vi "Optics_Open_COM.VI"(8 "Error in":errorcluster, 11 "VISA in":refnum<visa-resource-name>) -> (0 "Error out":errorcluster, 3 "VISA out":refnum<visa-resource-name>)   [LabVIEW 2021]
uses:
  <vilib>/Instr/_visa.llb/VISA Configure Serial Port (Instr).vi
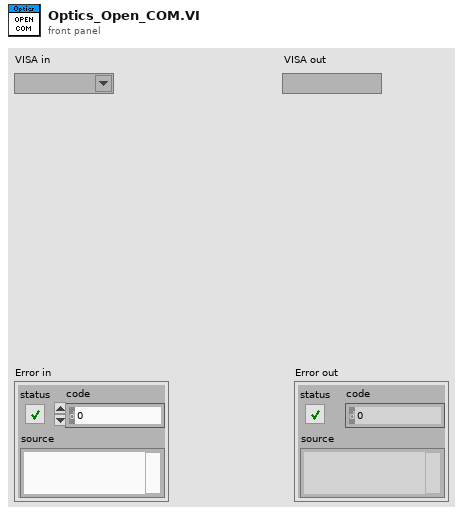
[diagram p1: front panel]
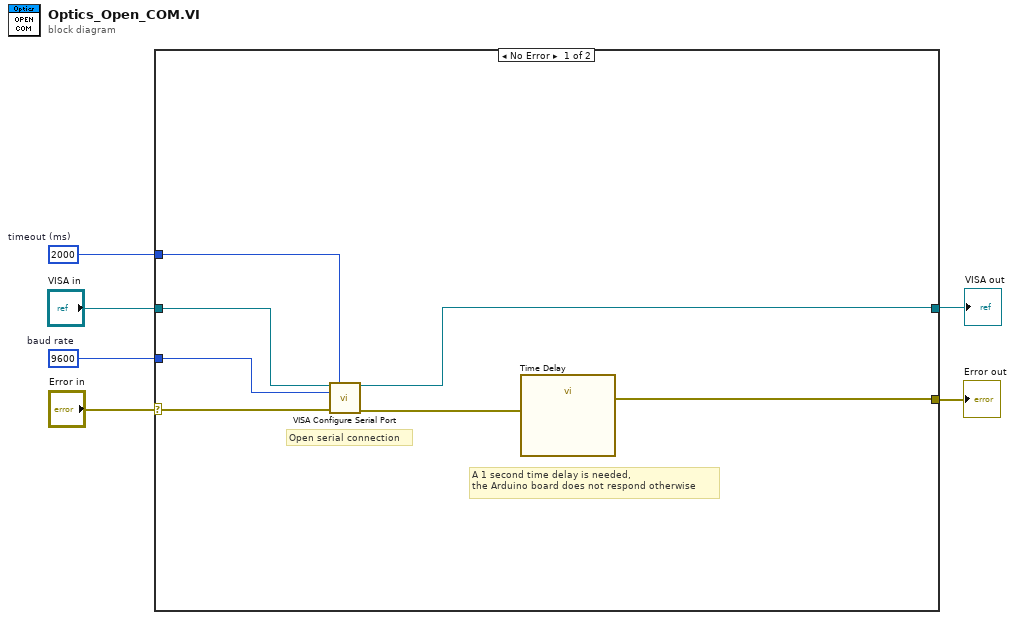
[diagram p0: block diagram]
diagram:
  w2 = u32 9600  # baud rate
  w1 = 2000  # timeout (ms)
  n1 = case shown="No Error" "Error in" {
    selector: "Error in" -> [w13 w15]
    tunnel: [w11 w15] -> w6
    tunnel: [w10 w14] -> w4
    tunnel: "VISA in" -> [w9 w14]
    tunnel: w2 -> [w8 _]
    tunnel: w1 -> [w7 _]
    frame No Error {
      # "Open serial connection"
      # "A 1 second time delay is needed, \nthe Arduino board does not respond otherwise"
      n2 = call-poly "VISA Configure Serial Port"("VISA resource name"=w9, "timeout (10sec)"=w7, "baud rate (9600)"=w8, "error in (no error)"=w13) -> ("VISA resource name out"=w10:refnum<visa-resource-name>, "error out"=w12:errorcluster)  [unwired: 10 in]
      n3 = call "Time Delay"("error in (no error)"=w12) -> ("error out"=w11:errorcluster)  [unwired: 10 in]
    }
    frame Default {
    }
  }
  "Error out" <- w6
  "VISA out" <- w4
